vi "eyeballT.vi"() -> ()   [LabVIEW 2018]
panel:
  in  "Numeric":i32
  out "error out":errorcluster
  in  "milliseconds to wait":u32
  out "Numeric 2":i32
  in  "stop":bool
  in  "error in (no error)":errorcluster
  in  "Python version":string="3.6"
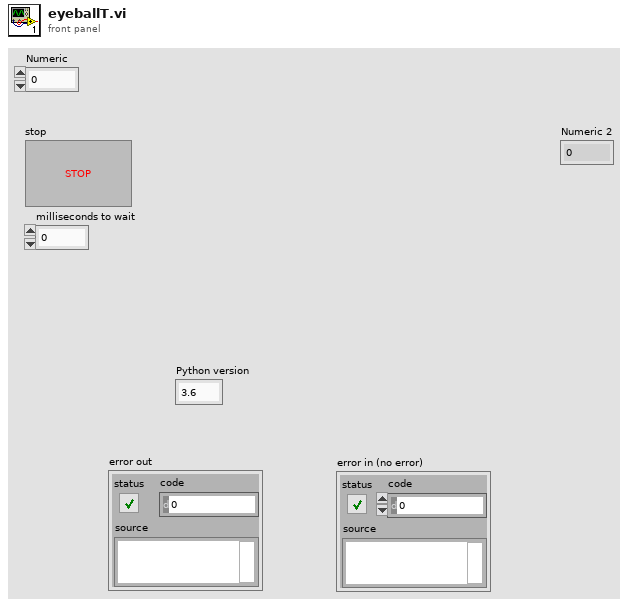
[diagram p1: front panel]
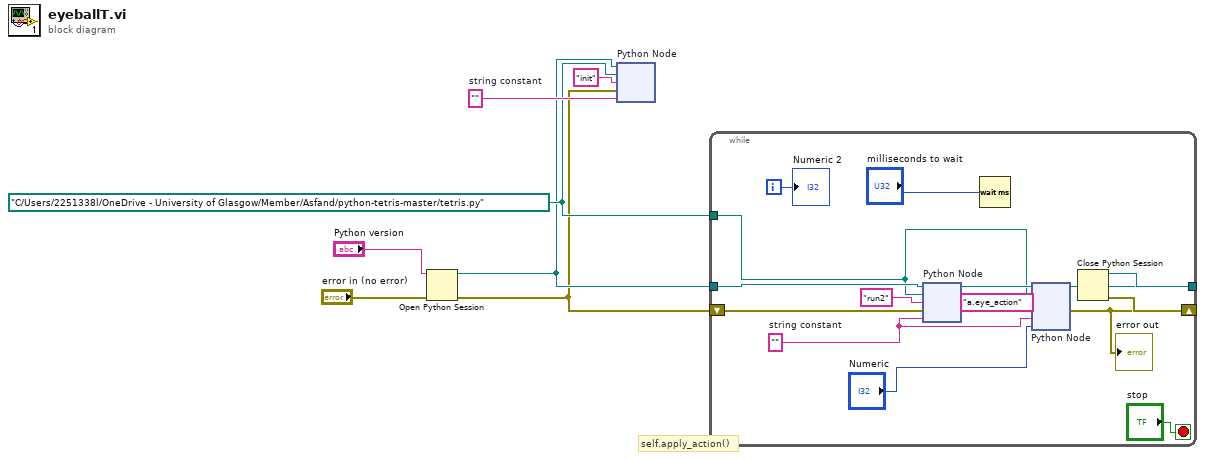
[diagram p0: block diagram]
diagram:
  w5 = path "C:/Users/2251338l/OneDrive - University of Glasgow/Member/Asfand/python-tetris-master/tetris.py" ("module path")
  w6 = ""  # string constant
  # "self.apply_action()"
  n1 = Open Python Session(python version="Python version", 3:"error in (no error)") -> (session out=w2:refnum<k35>, error out=w1:errorcluster)  [unwired: 1 in]
  n2 = node "Python Node"(w2, w5, "init" ("function name"), w1, w6) -> ()  [unwired: 1 in, 4 out]
  n3 = while {
    shift-right: [w17] -> w3
    shift-left: w1 -> [w22]
    tunnel: w2 -> [w21]
    tunnel: w5 -> [w13]
    tunnel: [w15] -> w4
    i -> [w19]
    stop <- "stop" stop-if-true
    w14 = ""  # string constant
    n4 = node "Python Node"(w21, w13, "run2" ("function name"), w22, w14) -> (w16:refnum<k35>, w18:errorcluster)  [unwired: 1 in, 2 out]
    n5 = Wait (ms)(milliseconds to wait="milliseconds to wait") -> ()  [unwired: 1 out]
    n6 = node "Python Node"(w16, w13, "a.eye_action" ("function name"), w18, w14, "Numeric") -> (w15:refnum<k35>, w17:errorcluster)  [unwired: 2 in, 2 out]
    "error out" <- w17
    "Numeric 2" <- w19
  }
  n7 = Close Python Session(session in=w4, error in=w3) -> ()  [unwired: 1 out]
